vi "Estimation_Steps.vi"(7 "Target(degree)":dbl format="%#_13g", 9 "Source_Phase_Step":i32, 11 "Input_Phase(degree)":dbl format="%#_13g") -> (1 "diff.Steps":i32, 3 "Esitmation_Step":i32)   [LabVIEW 2023, in "HAPS.lvlib"]
uses:
  HAPS.lvlib
panel:
  out "diff.Steps(DBL)":dbl
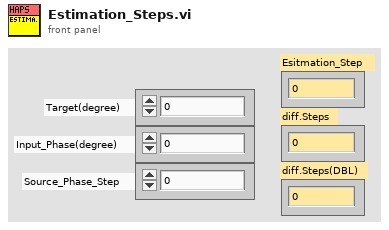
[diagram p1: front panel]
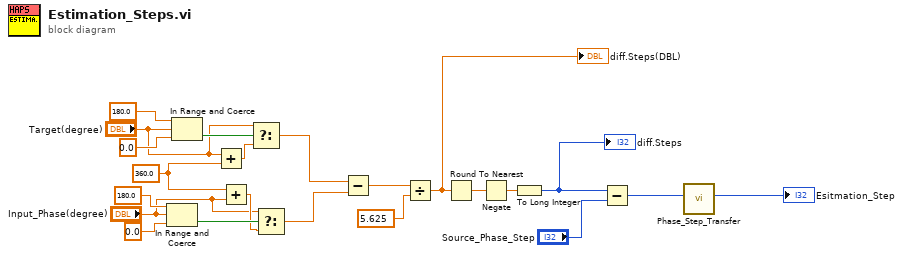
[diagram p0: block diagram]
diagram:
  w12 = 360.0 ("y")
  n1 = In Range and Coerce(upper limit=180.0, x="Input_Phase(degree)", lower limit=0.0) -> (In Range?=w11:bool)  [unwired: 1 out]
  n2 = In Range and Coerce(upper limit=180.0, x="Target(degree)", lower limit=0.0) -> (In Range?=w13:bool)  [unwired: 1 out]
  n3 = Add(x="Target(degree)", y=w12) -> (x+y=w9:dbl)
  n4 = Add(x=w12, y="Input_Phase(degree)") -> (x+y=w10:dbl)
  n5 = Select(t="Target(degree)", s=w13, f=w9) -> (s? t:f=w6:dbl)
  n6 = Select(t="Input_Phase(degree)", s=w11, f=w10) -> (s? t:f=w5:dbl)
  n7 = Subtract(x=w6, y=w5) -> (x-y=w22:dbl)
  n8 = Divide(x=w22, y=5.625) -> (x/y=w18:dbl)
  "diff.Steps(DBL)" <- w18
  n9 = Round To Nearest(number=w18) -> (nearest integer value=w19:dbl)
  n10 = Negate(x=w19) -> (-x=w3:dbl)
  n11 = To Long Integer(number=w3) -> (32bit integer=w2:i32)
  "diff.Steps" <- w2
  n12 = Subtract(x=w2, y="Source_Phase_Step") -> (x-y=w4:i32)
  n13 = call "Phase_Step_Transfer.vi"("Input_Phase_Step"=w4) -> ("Output_Phase_Step"=→"Esitmation_Step":i32)  [unwired: 10 in]
